vi "Test Multiple Doors API.vi"() -> ()   [LabVIEW 2018]
uses:
  Timed Door.lvclass
  Door/Door.lvclass
  Timed Door.lvclass/Timed Door.ctl
  Set Door.vi
  Set Target Time (seconds).vi
panel:
  out "error out":errorcluster
  in  "Create New Door":bool
  in  "Door Type":enum32{"Door", "Timed Door"}(radio)
  in  "Timed Door Target Time (seconds)":dbl=5.0
  in  "Door Switches":enum32{"Open Door", "Close Door"}[](array[radio])
  out "Door":u16[](array[ring])
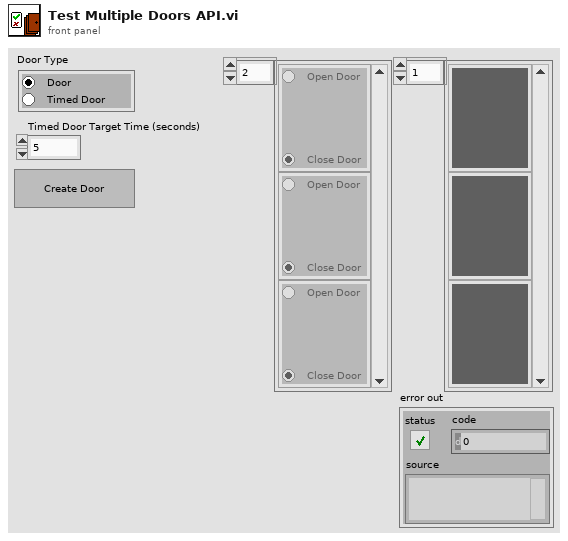
[diagram p1: front panel]
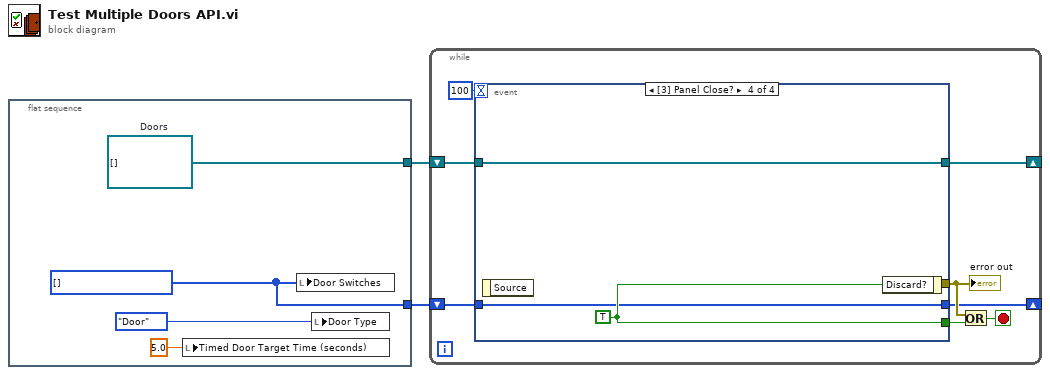
[diagram p0: block diagram]
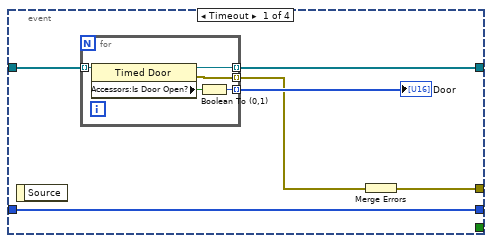
[diagram p2: hidden frame]
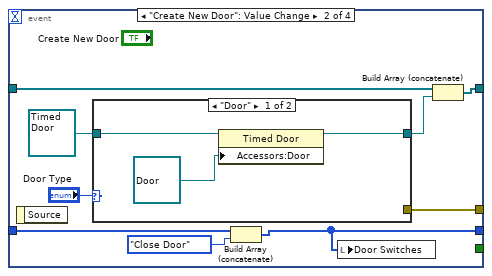
[diagram p3: hidden frame]
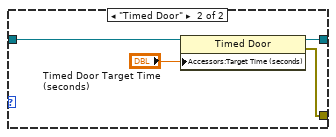
[diagram p4: hidden frame]
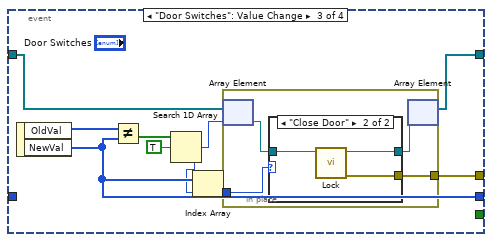
[diagram p5: hidden frame]
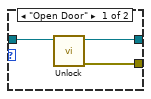
[diagram p6: hidden frame]
diagram:
  n1 = flat-sequence {
    tunnel: [w6] -> w2
    tunnel: [w3] -> w1
    frame #0 {
      w6 = refnum<class "Timed Door.lvclass">[] []  # Doors
      w3 = enum32{"Open Door", "Close Door"}[] [] items=["Open Door", "Close Door"] ("Door Switch")
      n2 = local write "Timed Door Target Time (seconds)"(5.0 ("Timed Door Target Time (seconds)")) -> ()
      n3 = local write "Door Switches"(w3) -> ()
      n4 = local write "Door Type"(enum32{"Door", "Timed Door"}."Door" ("Door Type")) -> ()
    }
  }
  n5 = while {
    shift-right: [w10] -> _
    shift-left: w2 -> [w12]
    shift-right: [w8] -> _
    shift-left: w1 -> [w9]
    stop <- w7 stop-if-true
    n6 = event shown="[3] Panel Close?" {
      selector: _ -> [_ _ _ _]
      dyn-events: _ -> [_ _ _ _]
      timeout: 100 -> [_ _ _ _]
      tunnel: w12 -> [w18 w34 w46 w62]
      tunnel: [_ _ _ w63] -> w11
      tunnel: [w19 w33 w47 w62] -> w10
      tunnel: w9 -> [w17 w30 _ w61]
      tunnel: [w17 w28 w45 w61] -> w8
      tunnel: [w15 w27 w42 _] -> w14
      event Timeout {
        n7 = event-data() -> ()  [unwired: 1 in, 1 out]
        n8 = for {
          tunnel: [w24] -> w20 mode=indexing
          tunnel: [w23] -> w19 mode=indexing
          tunnel: w18 -> [w22] mode=indexing
          tunnel: [w21] -> w16 mode=indexing
          n9 = property class="Timed Door"(reference=w22) -> (reference out=w23:refnum<class "Timed Door.lvclass">, error out=w21:errorcluster, "Accessors:Is Door Open?"=w25:bool)  [unwired: 1 in]
          n10 = Boolean To (0,1)(Boolean=w25) -> (0, 1=w24:i16)
        }
        "Door" <- w20
        n11 = Merge Errors(w16) -> (w15:errorcluster)
      }
      event "Create New Door": Value Change {
        n12 = event-data() -> ()  [unwired: 1 in, 1 out]
        n13 = case shown="\"Door\"" "Door Type" {
          tunnel: [w35 w41] -> w31
          tunnel: [_ w39] -> w27
          tunnel: refnum<class "Timed Door.lvclass"> refnum ("Timed Door.lvclass") -> [w37 w38]
          frame "Door" {
            n14 = property class="Timed Door"(reference=w37, "Accessors:Door"=refnum<class "Door.lvclass"> refnum ("Door")) -> (reference out=w35:refnum<class "Timed Door.lvclass">)  [unwired: 1 in, 1 out]
          }
          frame "Timed Door" {
            n15 = property class="Timed Door"(reference=w38, "Accessors:Target Time (seconds)"="Timed Door Target Time (seconds)") -> (reference out=w41:refnum<class "Timed Door.lvclass">, error out=w39:errorcluster)  [unwired: 1 in]
          }
        }
        n16 = Build Array (concatenate)(w30, enum32{"Open Door", "Close Door"}."Close Door" ("Door Switch")) -> (w28:enum32{"Open Door", "Close Door"}[])
        n17 = local write "Door Switches"(w28) -> ()
        n18 = Build Array (concatenate)(w34, w31) -> (w33:refnum<class "Timed Door.lvclass">[])
      }
      event "Door Switches": Value Change {
        n19 = event-data() -> ("OldVal"=w50:enum32{"Open Door", "Close Door"}[], "NewVal"=w45:enum32{"Open Door", "Close Door"}[])  [unwired: 1 in]
        n20 = Not Equal?(x=w50, y=w45) -> (x != y?=w49:bool[])
        n21 = Search 1D Array(1D array=w49, element=TRUE) -> (index of element=w44:i32)  [unwired: 1 in]
        n22 = Index Array(array=w45, index=w44) -> (element=w43:enum32{"Open Door", "Close Door"})
        n23 = in-place {
          in-place-border: w43 -> [w52]
          in-place-border: [w51] -> w42
          n24 = in-place-array #1(w46, w44) -> (w54:refnum<class "Timed Door.lvclass">)
          n25 = case shown="\"Close Door\"" w52 {
            tunnel: w54 -> [w57 w60]
            tunnel: [w56 w59] -> w53
            tunnel: [w55 w58] -> w51
            frame "Open Door" {
              n26 = call-dynamic "Unlock.vi"("Timed Door in"=w57) -> ("error out"=w55:errorcluster, "Timed Door out"=w56:refnum<class "Timed Door.lvclass">)  [unwired: 9 in]
            }
            frame "Close Door" {
              n27 = call-dynamic "Lock.vi"("Timed Door in"=w60) -> ("error out"=w58:errorcluster, "Timed Door out"=w59:refnum<class "Timed Door.lvclass">)  [unwired: 9 in]
            }
          }
          n28 = in-place-array #1(w53) -> (w47:refnum<class "Timed Door.lvclass">[])  [unwired: 1 out]
        }
      }
      event Panel Close? {
        w63 = TRUE ("Discard?")
        n29 = event-data() -> ()  [unwired: 1 in, 1 out]
        n30 = event-data("Discard?"=w63) -> ()  [unwired: 1 in, 1 out]
      }
    }
    "error out" <- w14
    n31 = Or(x=w14, y=w11) -> (x .or. y?=w7:bool)
  }
